vi "Select Pins to Publish by Device Type.vi"(8 "error in (no error)":errorcluster, 11 "USID":T1 max=15) -> (0 "error out":errorcluster, 3 "Pins_To_Publish":string[](array[string]))   [LabVIEW 2013]
uses:
  Controls/USID.ctl
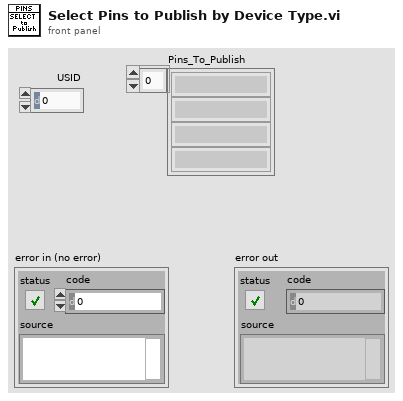
[diagram p1: front panel]
types:
  T1 = typedef "USID.ctl" = u8
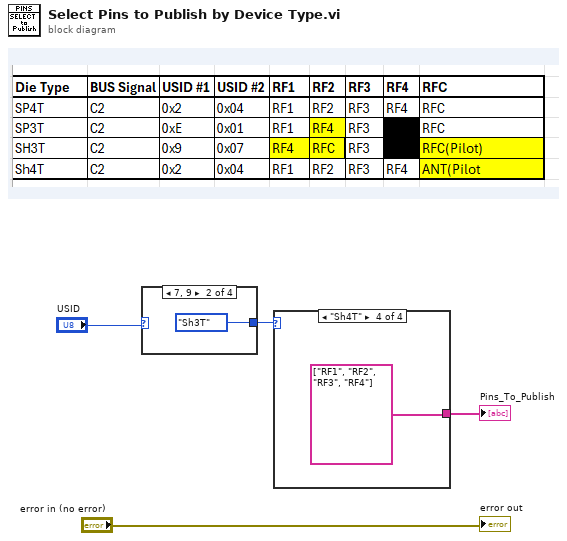
[diagram p0: block diagram]
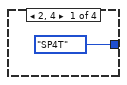
[diagram p2: hidden frame]
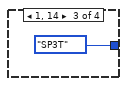
[diagram p3: hidden frame]
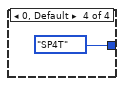
[diagram p4: hidden frame]
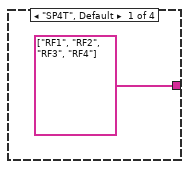
[diagram p5: hidden frame]
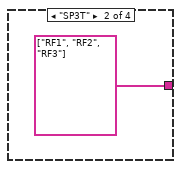
[diagram p6: hidden frame]
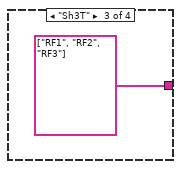
[diagram p7: hidden frame]
diagram:
  n1 = case shown="7, 9" "USID" {
    tunnel: [enum16{"SP4T", "SP3T", "Sh3T", "Sh4T"}."SP4T" ("Die Type 2") enum16{"SP4T", "SP3T", "Sh3T", "Sh4T"}."Sh3T" ("Die Type 2") enum16{"SP4T", "SP3T", "Sh3T", "Sh4T"}."SP3T" ("Die Type 2") enum16{"SP4T", "SP3T", "Sh3T", "Sh4T"}."SP4T" ("Die Type 2")] -> w2
    frame 2, 4 {
    }
    frame 7, 9 {
    }
    frame 1, 14 {
    }
    frame 0, Default {
    }
  }
  n2 = case shown="\"Sh4T\"" w2 {
    tunnel: [string[] ["RF1", "RF2", "RF3", "RF4"] ("Pins_To_Publish") string[] ["RF1", "RF2", "RF3"] ("Pins_To_Publish") string[] ["RF1", "RF2", "RF3"] ("Pins_To_Publish") string[] ["RF1", "RF2", "RF3", "RF4"] ("Pins_To_Publish")] -> w1
    frame "SP4T", Default {
    }
    frame "SP3T" {
    }
    frame "Sh3T" {
    }
    frame "Sh4T" {
    }
  }
  "Pins_To_Publish" <- w1
  "error out" <- "error in (no error)"
